vi "距离.vi"(1 "目前位置":cluster{"x（cm）":dbl, "y（cm）":dbl, "角度（度）":dbl}, 2 "目标位置":cluster{"x（cm）":dbl, "y（cm）":dbl, "角度（度）":dbl}) -> (0 "距离":dbl)   [LabVIEW 2016]
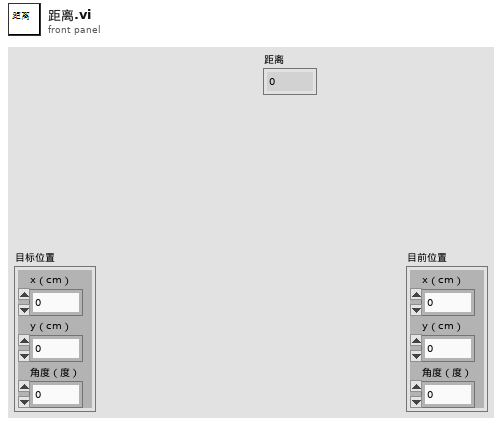
[diagram p1: front panel]
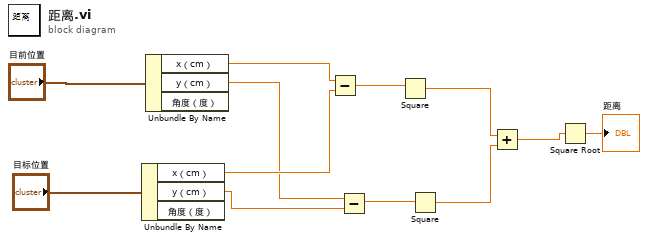
[diagram p0: block diagram]
diagram:
  n1 = Unbundle By Name("目标位置") -> ("x（cm）"=w9:dbl, "y（cm）"=w7:dbl)  [unwired: 1 out]
  n2 = Unbundle By Name("目前位置") -> ("x（cm）"=w10:dbl, "y（cm）"=w8:dbl)  [unwired: 1 out]
  n3 = Subtract(x=w10, y=w9) -> (x-y=w6:dbl)
  n4 = Subtract(x=w8, y=w7) -> (x-y=w5:dbl)
  n5 = Square(x=w6) -> (x^2=w4:dbl)
  n6 = Square(x=w5) -> (x^2=w3:dbl)
  n7 = Add(x=w4, y=w3) -> (x+y=w2:dbl)
  n8 = Square Root(x=w2) -> (sqrt(x)=→"距离":dbl)
